vi "Modfy TV Panel.vi"(8 "error in (no error)":errorcluster) -> (0 "error out":errorcluster)   [LabVIEW 2014]
uses:
  Type'def/FTT Display Type.ctl
panel:
  in  "Cancel":bool
  in  "Save":bool
  in  "modfy TV FTT":T1
  # "Modfy TV FTT"
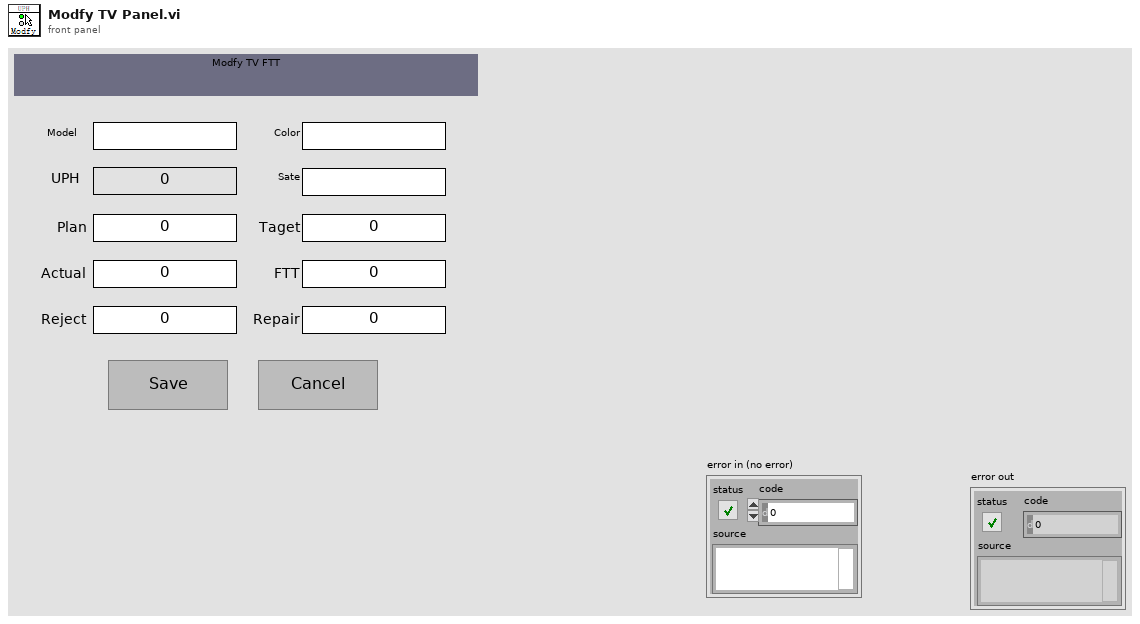
[diagram p1: front panel]
types:
  T1 = cluster{"Model":string, "Color":string, "UPH":dbl, "Sate":string, "Plan":dbl, "Taget":dbl, "Actual":dbl, "FTT":dbl, "Reject":dbl, "Repair":dbl}
  T2 = typedef "FTT Display Type.ctl" = cluster{"Line.No":string, "Model":string, "Color":string, "UPH":dbl, "Plan":dbl, "Target Rate":dbl, "Target ":dbl, "Actual":dbl, "FTT":dbl, "FTT Rate":dbl, "Repaired":dbl, "Reject":dbl, "Ouline":dbl, "Line State":string}
  T3 = cluster{"modfy TV FTT":cluster{"Model":string, "Color":string, "UPH":dbl, "Sate":string, "Plan":dbl, "Taget":dbl, "Actual":dbl, "FTT":dbl, "Reject":dbl, "Repair":dbl}, "Display":T2}
  T4 = cluster{"Display":T2, "Class":enum16{"Big", "Small"}}
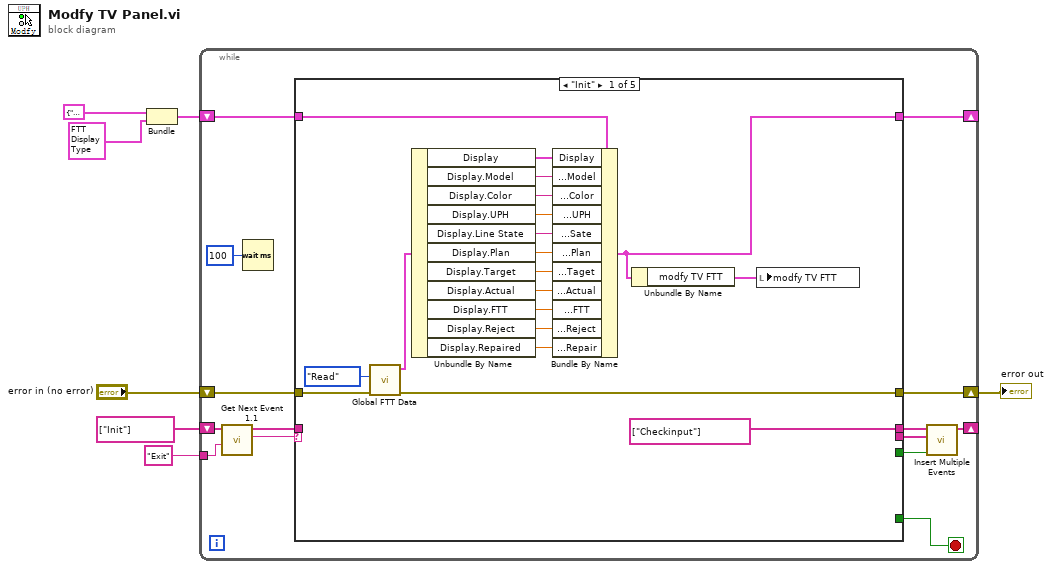
[diagram p0: block diagram]
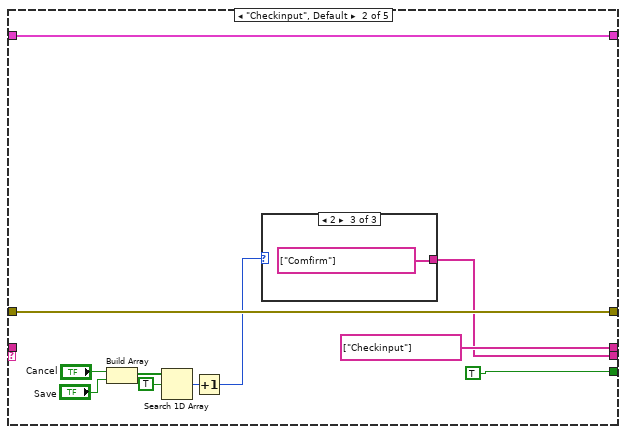
[diagram p2: hidden frame]
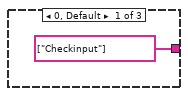
[diagram p3: hidden frame]
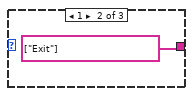
[diagram p4: hidden frame]
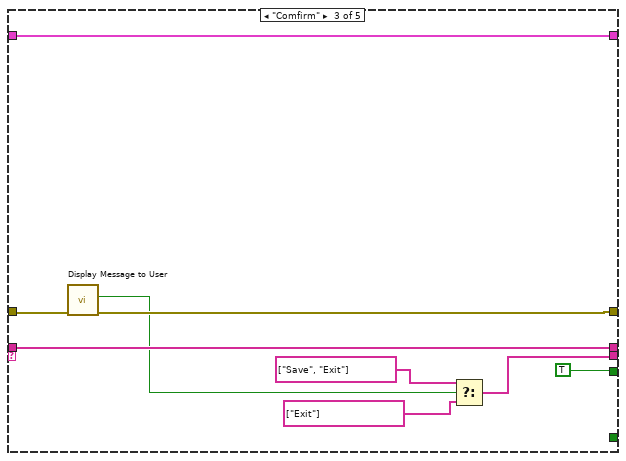
[diagram p5: hidden frame]
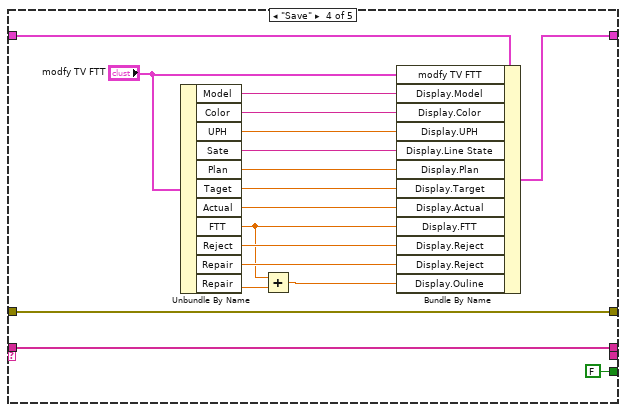
[diagram p6: hidden frame]
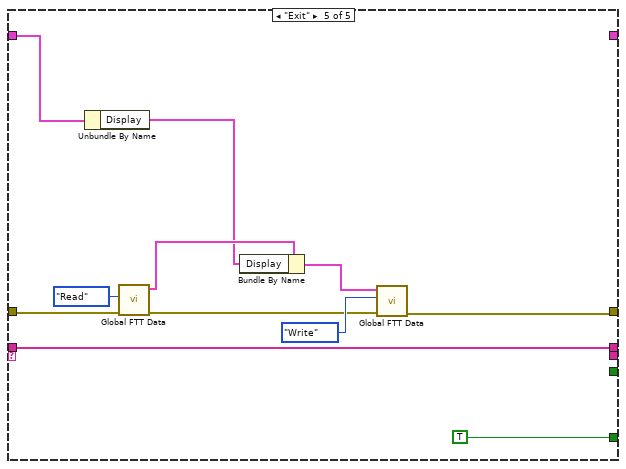
[diagram p7: hidden frame]
diagram:
  n1 = Bundle("modfy TV FTT"=T1 {"Model"="", "Color"="", "UPH"=0.0, "Sate"="", "Plan"=0.0, "Taget"=12.0, "Actual"=0.0, "FTT"=0.0, "Reject"=0.0, "Repair"=0.0}, "Display"=T2 {"Line.No"="", "Model"="", "Color"="", "UPH"=0.0, "Plan"=0.0, "Target Rate"=0.0, "Target "=0.0, "Actual"=0.0, "FTT"=0.0, "FTT Rate"=0.0, "Repaired"=0.0, "Reject"=0.0, "Ouline"=0.0, "Line State"=""}) -> (w3:T3)  [unwired: 1 in]
  n2 = while {
    tunnel: "Exit" ("Exit Event") -> [w17]
    shift-right: [w14] -> w1
    shift-left: "error in (no error)" -> [w16]
    shift-right: [w10] -> _
    shift-left: w3 -> [w15]
    shift-right: [w13] -> _
    shift-left: string[] ["Init"] -> [w19]
    stop <- w8 stop-if-true
    n3 = call "Get Next Event 1.1.vi"("Exit Event"=w17, "event queue in"=w19) -> ("next event"=w20:string, "event queue out"=w18:string[])  [unwired: 6 in, 2 out]
    n4 = Wait (ms)(milliseconds to wait=u32 100) -> ()  [unwired: 1 out]
    n5 = case shown="\"Init\"" w20 {
      tunnel: w18 -> [_ _ w62 w80 w91]
      tunnel: w16 -> [w40 w51 w61 w81 w87]
      tunnel: w15 -> [w36 w42 w63 w79 w88]
      tunnel: [w38 w51 w60 w81 w90] -> w14
      tunnel: [string[] ["Checkinput"] string[] ["Checkinput"] w62 w80 w91] -> w12
      tunnel: [_ TRUE TRUE FALSE _] -> w11
      tunnel: [w24 w42 w63 w78 _] -> w10
      tunnel: [_ w41 w55 _ _] -> w9
      tunnel: [_ _ _ _ TRUE] -> w8
      frame "Init" {
        n6 = call "Global FTT Data.vi"("error in (no error)"=w40, "Mode"=enum16{"Read", "Write"}."Read") -> ("error out"=w38:errorcluster, "Cluster"=w35:T4)  [unwired: 8 in]
        n7 = Unbundle By Name(w35) -> ("Display"=w22:T2, "Display.Model"=w34:string, "Display.Color"=w33:string, "Display.UPH"=w32:dbl, "Display.Line State"=w31:string, "Display.Plan"=w30:dbl, "Display.Target"=w29:dbl, "Display.Actual"=w28:dbl, "Display.FTT"=w27:dbl, "Display.Reject"=w26:dbl, "Display.Repaired"=w25:dbl)
        n8 = Bundle By Name(cluster=w36, "Display"=w22, "modfy TV FTT.Model"=w34, "modfy TV FTT.Color"=w33, "modfy TV FTT.UPH"=w32, "modfy TV FTT.Sate"=w31, "modfy TV FTT.Plan"=w30, "modfy TV FTT.Taget"=w29, "modfy TV FTT.Actual"=w28, "modfy TV FTT.FTT"=w27, "modfy TV FTT.Reject"=w26, "modfy TV FTT.Repair"=w25) -> (w24:T3)
        n9 = Unbundle By Name(w24) -> ("modfy TV FTT"=w23:T1)
        n10 = local write "modfy TV FTT"(w23) -> ()
      }
      frame "Checkinput", Default {
        n11 = Build Array("Cancel", "Save") -> (w47:bool[])
        n12 = Search 1D Array(1D array=w47, element=TRUE) -> (index of element=w45:i32)  [unwired: 1 in]
        n13 = Increment(x=w45) -> (x+1=w43:i32)
        n14 = case shown="2" w43 {
          tunnel: [string[] ["Checkinput"] string[] ["Exit"] string[] ["Comfirm"]] -> w41
          frame 0, Default {
          }
          frame 1 {
          }
          frame 2 {
          }
        }
      }
      frame "Comfirm" {
        n15 = call "Display Message to User"("error in (no error)"=w61) -> ("error out"=w60:errorcluster, "OK"=w58:bool)  [unwired: 9 in]
        n16 = Select(t=string[] ["Save", "Exit"], s=w58, f=string[] ["Exit"]) -> (s? t:f=w55:string[])
      }
      frame "Save" {
        n17 = Unbundle By Name("modfy TV FTT") -> ("Model"=w76:string, "Color"=w75:string, "UPH"=w74:dbl, "Sate"=w73:string, "Plan"=w72:dbl, "Taget"=w71:dbl, "Actual"=w70:dbl, "FTT"=w65:dbl, "Reject"=w69:dbl, "Repair"=w68:dbl, "Repair"=w66:dbl)
        n18 = Add(x=w65, y=w66) -> (x+y=w64:dbl)
        n19 = Bundle By Name(cluster=w79, "modfy TV FTT"="modfy TV FTT", "Display.Model"=w76, "Display.Color"=w75, "Display.UPH"=w74, "Display.Line State"=w73, "Display.Plan"=w72, "Display.Target"=w71, "Display.Actual"=w70, "Display.FTT"=w65, "Display.Reject"=w69, "Display.Reject"=w68, "Display.Ouline"=w64) -> (w78:T3)
      }
      frame "Exit" {
        n20 = Unbundle By Name(w88) -> ("Display"=w83:T2)
        n21 = call "Global FTT Data.vi"("error in (no error)"=w87, "Mode"=enum16{"Read", "Write"}."Read") -> ("error out"=w86:errorcluster, "Cluster"=w84:T4)  [unwired: 8 in]
        n22 = Bundle By Name(cluster=w84, "Display"=w83) -> (w82:T4)
        n23 = call "Global FTT Data.vi"("error in (no error)"=w86, "Mode"=enum16{"Read", "Write"}."Write", "Display"=w82) -> ("error out"=w90:errorcluster)  [unwired: 7 in, 1 out]
      }
    }
    n24 = call "Insert Multiple Events.vi"("Insert all? (T)"=w11, "Events to Insert"=w9, "Event queue in"=w12) -> ("Event queue out"=w13:string[])  [unwired: 4 in]
  }
  "error out" <- w1
